vi "Find Dynamic Test Methods.vi"(7 "Test Case class name":string, 8 "error in (no error)":errorcluster, 10 "Test Methods In":map{string, path}(c390), 11 "LVClassLibrary in":refnum<vi>) -> (0 "error out":errorcluster, 2 "Test Methods Out":map{string, path}(c390), 3 "LVClassLibrary out":refnum<vi>)   [LabVIEW 2020, in "Test Finder.lvclass"]
uses:
  Test Finder.lvclass
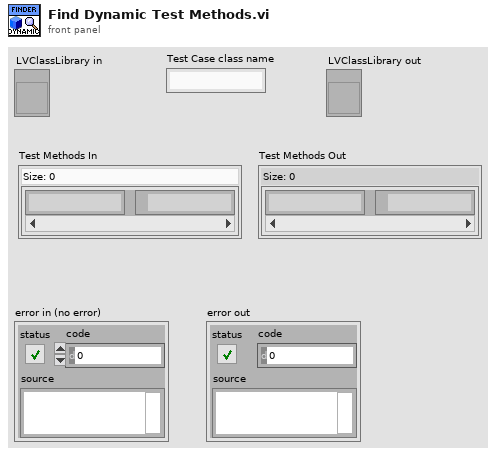
[diagram p1: front panel]
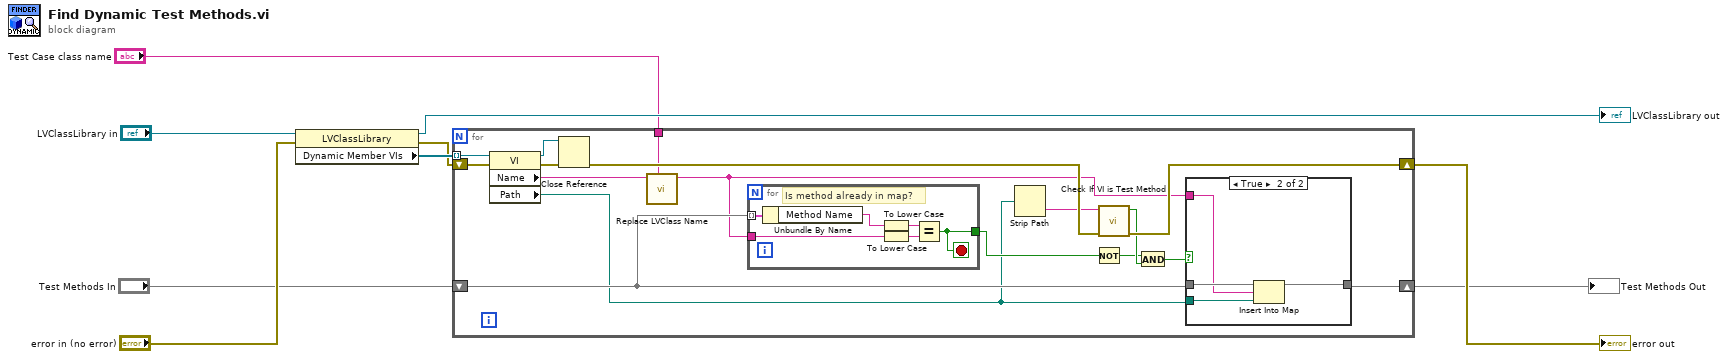
[diagram p0: block diagram]
diagram:
  n1 = property class="LVClassLibrary"(reference="LVClassLibrary in", error in="error in (no error)") -> (reference out=→"LVClassLibrary out":refnum<vi>, error out=w5:errorcluster, "Dynamic Member VIs"=w6:refnum<vi>[])
  n2 = for {
    tunnel: w6 -> [w24] mode=indexing
    shift-right: [w19] -> w4
    shift-left: w5 -> [w23]
    shift-right: [w20] -> w2
    shift-left: "Test Methods In" -> [w21]
    tunnel: "Test Case class name" -> [w13]
    n3 = property class="VI"(reference=w24, error in=w23) -> (reference out=w26:refnum<vi>, error out=w25:errorcluster, "Name"=w14:string, "Path"=w11:path)
    n4 = Close Reference(reference=w26, error in (no error)=w25) -> (error out=w16:errorcluster)
    n5 = call "Replace LVClass Name.vi"("Test Case class name"=w13, "Name in"=w14) -> ("Name out"=w15:string)  [unwired: 9 in]
    n6 = for {
      tunnel: [w27] -> w22
      tunnel: w21 -> [w32] mode=indexing
      tunnel: w15 -> [w28]
      stop <- w27 stop-if-true
      # "Is method already in map?"
      n7 = Unbundle By Name(w32) -> ("Method Name"=w30:string)
      n8 = To Lower Case(string=w30) -> (all lower case string=w31:string)
      n9 = To Lower Case(string=w28) -> (all lower case string=w29:string)
      n10 = Equal?(x=w31, y=w29) -> (x = y?=w27:bool)
    }
    n11 = Strip Path(path=w11) -> (name=w10:string)  [unwired: 1 out]
    n12 = Not(x=w22) -> (.not. x?=w12:bool)
    n13 = call "Check If VI is Test Method.vi"("error in (no error)"=w16, "VI Name"=w10) -> ("error out"=w19:errorcluster, "Is Test Method?"=w17:bool)  [unwired: 8 in]
    n14 = And(x=w12, y=w17) -> (x .and. y?=w18:bool)
    n15 = case shown="True" w18 {
      tunnel: w21 -> [w33 w37]
      tunnel: w15 -> [_ w36]
      tunnel: w11 -> [_ w35]
      tunnel: [w33 w34] -> w20
      frame False {
        # "When finding dynamic methods we allways keep the one closest in the class hirarchy"
      }
      frame True {
        n16 = Insert Into Map(map in=w37, key=w36, value=w35) -> (map out=w34:map{string, path})  [unwired: 2 out]
      }
    }
  }
  "error out" <- w4
  "Test Methods Out" <- w2
